vi "RunTestVi.vi"   [LabVIEW 2020]
uses:
  _ContextHelp Editor/ContextHelpEditor.lvlib
panel:
  # "QuickDropTester"
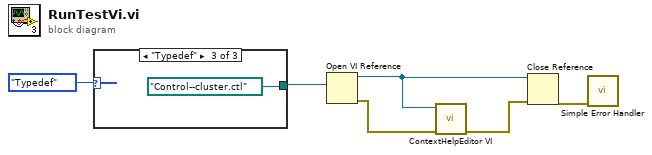
[diagram p0: block diagram]
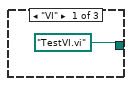
[diagram p2: hidden frame]
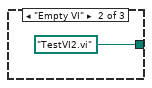
[diagram p3: hidden frame]
diagram:
  n1 = case shown="\"Typedef\"" enum16{"VI", "Empty VI", "Typedef"}."Typedef" {
    tunnel: [path "TestVI.vi" ("vi path") path "TestVI2.vi" ("vi path") path "Control--cluster.ctl" ("vi path")] -> w2
    frame "VI" {
    }
    frame "Empty VI" {
    }
    frame "Typedef" {
    }
  }
  n2 = Open VI Reference(vi path=w2) -> (vi reference=w4:refnum<vi>, error out=w6:errorcluster)  [unwired: 5 in]
  n3 = call "ContextHelpEditor VI.vi"("error in (no error)"=w6, "VI Ref"=w4) -> ("error out"=w5:errorcluster)  [unwired: 9 in]
  n4 = Close Reference(reference=w4, error in (no error)=w5) -> (error out=w1:errorcluster)
  n5 = call <vilib>:"Simple Error Handler.vi"("error in (no error)"=w1) -> ()  [unwired: 4 in, 5 out]
